vi "AMZ_S3_APIHLP_Parse PUT Object ACL Result.vi"(8 "error in (no error)":errorcluster, 11 "Response header":string) -> (0 "error out":errorcluster, 3 "PutObjectACLResult":T1)   [LabVIEW 2015, in "LV Interface for Amazon S3.lvlib"]
uses:
  LV Interface for Amazon S3.lvlib
  Typedefs/AMZ_S3_API_PUTObjectACLResult.ctl
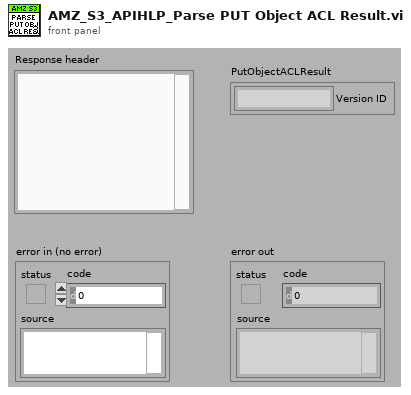
[diagram p1: front panel]
types:
  T1 = typedef "LV Interface for Amazon S3.lvlib/AMZ_S3_API_PUTObjectACLResult.ctl" = cluster{"Version ID":string}
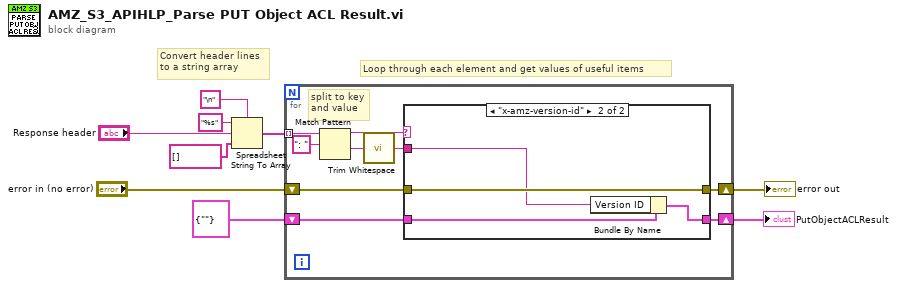
[diagram p0: block diagram]
diagram:
  # "Loop through each element and get values of useful items"
  # "Convert header lines\nto a string array"
  n1 = Spreadsheet String To Array(delimiter (Tab)="\n", format string="%s", spreadsheet string="Response header", array type (2D Dbl)=string[] []) -> (array=w6:string[])
  n2 = for {
    tunnel: w6 -> [w18] mode=indexing
    shift-right: [w14] -> w2
    shift-left: "error in (no error)" -> [w15]
    shift-right: [w12] -> w1
    shift-left: T1 {"Version ID"=""} ("PutObjectACLResult") -> [w13]
    # "split to key\nand value"
    n3 = Match Pattern(string=w18, regular expression=": ") -> (before substring=w16:string, after substring=w11:string)  [unwired: 1 in, 2 out]
    n4 = call <vilib>:"Trim Whitespace.vi"("string"=w11) -> ("trimmed string"=w10:string)  [unwired: 1 in]
    n5 = case shown="\"x-amz-version-id\"" w16 {
      tunnel: [w20 w22] -> w14
      tunnel: w15 -> [w20 w22]
      tunnel: w10 -> [_ w21]
      tunnel: w13 -> [w19 w24]
      tunnel: [w19 w23] -> w12
      frame Default {
      }
      frame "x-amz-version-id" {
        n6 = Bundle By Name(cluster=w24, "Version ID"=w21) -> (w23:T1)
      }
    }
  }
  "PutObjectACLResult" <- w1
  "error out" <- w2
